vi "OSC_PreSet.vi"(0 "resource name":refnum<k15>="PXI1Slot5" caption="Resource Name", 1 "vertical range":dbl=10.0 caption="Vertical Range (V)" format="%.2f", 5 "channel name":string="0" caption="Channel Name(s)", 7 "probe attenuation":dbl=10.0 caption="Probe Attenuation" format="%.1f", 9 "trigger source":string(combo)="0" caption="Trigger Source", 11 "reference position":dbl=50.0 caption="Ref Position" format="%.1f", 12 "trigger level":dbl=0.1 caption="Trigger Level" format="%.2f", 13 "trigger slope":T3 caption="Trigger Slope", 14 "min record length":i32=100 caption="Min. Record Length") -> (4 "instrument handle out":refnum<k15>, 6 "error out":errorcluster)   [LabVIEW 2013]
uses:
  <instrlib>/niScope/Controls/niScope trigger slope.ctl
  <instrlib>/niScope/Controls/niScope trigger coupling.ctl
  <instrlib>/niScope/Controls/niScope vertical coupling.ctl
  <instrlib>/niScope/Configure/Trigger/niScope Configure Trigger Edge.vi
panel:
  in  "enforce realtime":bool=TRUE caption="Enforce Realtime"
  in  "min sample rate":dbl=125000000.0 caption="Min. Sample Rate" step=1000000.0 format="%.2p"
  in  "vertical offset":dbl caption="Vertical Offset" format="%.4f"
  in  "input impedance":u32(ring) caption="Input Impedance" items=["1 mega ohm"=0, "50 ohms"=2]
  in  "maximum input frequency":dbl=125000000.0 caption="Max. Input Frequency" format="%.2p"
  in  "trigger delay":dbl caption="Trigger Delay" format="%.4p"
  in  "vertical coupling":T1=1 caption="Vertical Coupling" items=["AC", "DC", "Ground"]
  in  "trigger coupling":T2=1 caption="Trigger Coupling" items=["AC"=0, "DC"=1, "HF Reject"=3, "LF Reject"=4, "AC Plus HF Reject"=1001]
  in  "trigger modifier":i32(ring)=1 caption="Trigger Modifier" items=["None"=1, "Auto Trigger"=2]
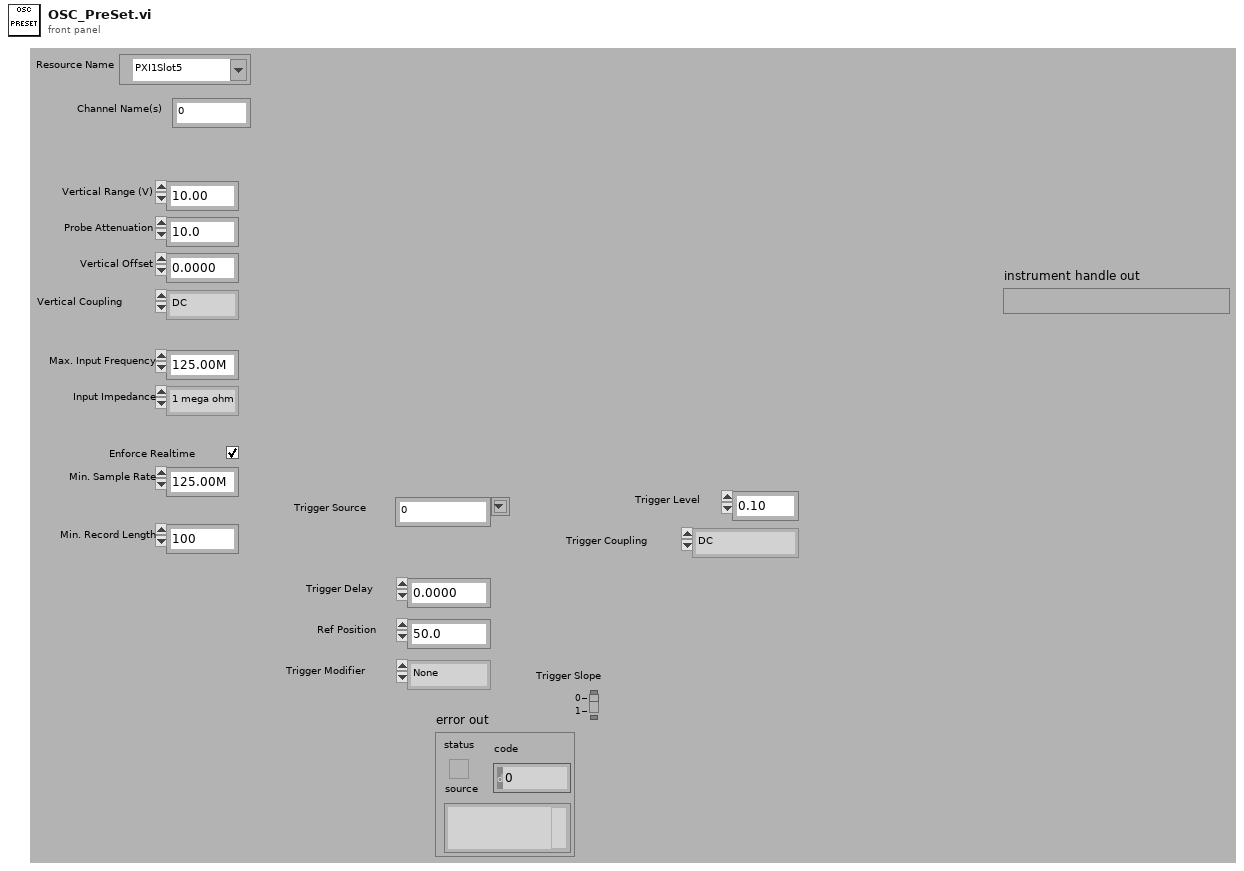
[diagram p1: front panel]
types:
  T1 = typedef "niScope vertical coupling.ctl" = i32
  T2 = typedef "niScope trigger coupling.ctl" = u16
  T3 = typedef "niScope trigger slope.ctl" = i32
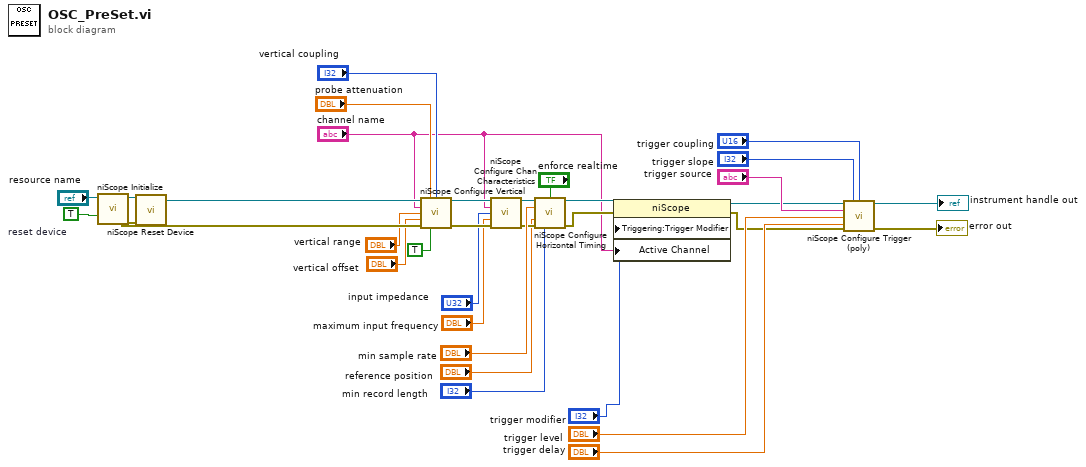
[diagram p0: block diagram]
diagram:
  w34 = TRUE  # reset device
  n1 = call <instrlib>:"niScope Initialize.vi"("resource name"="resource name", "reset device"=w34) -> ("instrument handle"=w29:refnum<k15>, "error out"=w30:errorcluster)  [unwired: 12 in]
  n2 = call <instrlib>:"niScope Reset Device.vi"("instrument handle"=w29, "error in"=w30) -> ("instrument handle out"=w31:refnum<k15>, "error out"=w32:errorcluster)  [unwired: 12 in]
  n3 = call <instrlib>:"niScope Configure Vertical.vi"("instrument handle"=w31, "probe attenuation"="probe attenuation", "vertical coupling"="vertical coupling", "channels"="channel name", "vertical range"="vertical range", "vertical offset"="vertical offset", "error in"=w32, "channel enabled"=TRUE) -> ("instrument handle out"=w25:refnum<k15>, "error out"=w24:errorcluster)  [unwired: 6 in]
  n4 = call <instrlib>:"niScope Configure Chan Characteristics.vi"("instrument handle"=w25, "channels"="channel name", "input impedance"="input impedance", "maximum input frequency"="maximum input frequency", "error in"=w24) -> ("instrument handle out"=w22:refnum<k15>, "error out"=w23:errorcluster)  [unwired: 9 in]
  n5 = call <instrlib>:"niScope Configure Horizontal Timing.vi"("instrument handle"=w22, "enforce realtime"="enforce realtime", "min sample rate"="min sample rate", "reference position"="reference position", "error in"=w23, "min record length"="min record length") -> ("instrument handle out"=w11:refnum<k15>, "error out"=w10:errorcluster)  [unwired: 8 in]
  n6 = property class="niScope"(reference=w11, error in=w10, "Triggering:Trigger Modifier"="trigger modifier", "Active Channel"="channel name") -> (reference out=w8:refnum<k15>, error out=w9:errorcluster)
  n7 = call-poly <instrlib>:"niScope Configure Trigger (poly).vi"("instrument handle"=w8, "trigger slope"="trigger slope", "trigger coupling"="trigger coupling", "trigger source"="trigger source", "trigger level"="trigger level", "error in"=w9, "trigger delay"="trigger delay") -> ("instrument handle out"=→"instrument handle out":refnum<k15>, "error out"=→"error out":errorcluster)  [unwired: 7 in]
